vi "Create Beam.vi"(8 "error in (no error)":errorcluster, 11 "XRay Beam in":refnum<class "XRay Beam.lvclass">) -> (0 "error out":errorcluster, 3 "XRay Beam out":refnum<class "XRay Beam.lvclass">)   [LabVIEW 2026, in "XRay Beam.lvclass"]
uses:
  XRay Beam.lvclass
  XRay Beam.lvclass/XRay Beam.ctl
  <vilib>/picture/3D Picture Control/Object/Create Object (name).vi
  <vilib>/picture/3D Picture Control/NI_3D Picture Control.lvlib
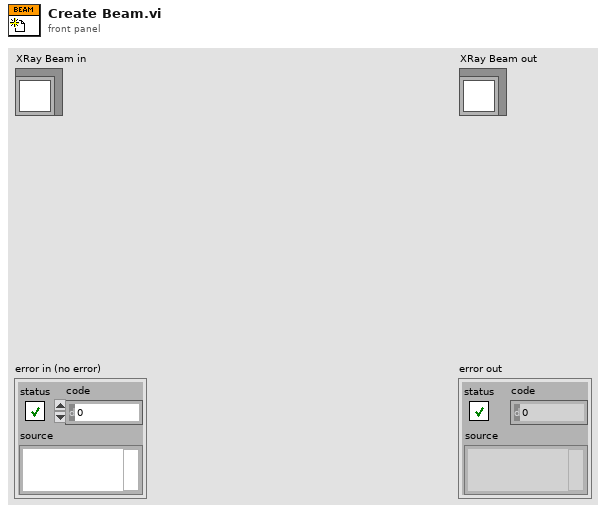
[diagram p1: front panel]
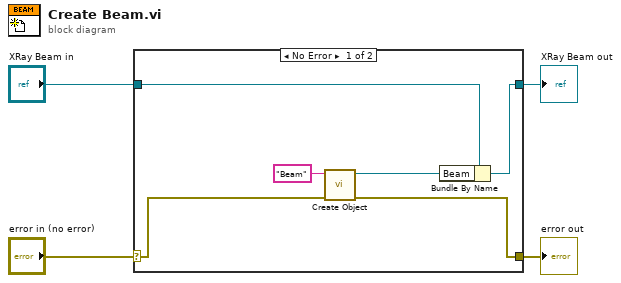
[diagram p0: block diagram]
diagram:
  n1 = case shown="No Error" "error in (no error)" {
    selector: "error in (no error)" -> [w6 w11]
    tunnel: [w5 w11] -> w3
    tunnel: [w9 w12] -> w1
    tunnel: "XRay Beam in" -> [w10 w12]
    frame No Error {
      n2 = call-poly <vilib>:"Create Object.vi"("error in (no error)"=w6, "Name"="Beam") -> ("error out"=w5:errorcluster, "Scene:New Object"=w7:refnum<vi>)  [unwired: 8 in]
      n3 = Bundle By Name(cluster=w10, "Beam"=w7) -> (w9:refnum<class "XRay Beam.lvclass">)
    }
    frame Error {
    }
  }
  "error out" <- w3
  "XRay Beam out" <- w1
